vi "Get Ethernet Configuration.vi"(8 "error in (no error)":errorcluster, 11 "Ethernet in":refnum<class "ENET_BS120x.lvclass">) -> (0 "error out":errorcluster, 1 "Configuration Error?":bool, 2 "Ethernet Settings":T1, 3 "Ethernet out":refnum<class "ENET_BS120x.lvclass">)   [LabVIEW 2021, in "BS120x Driver.lvlib" / "ENET_BS120x.lvclass"]
doc: "Retrieve Battery Simulator 1200 Ethernet settings.\n(c) 2019 Bloomy Controls, Inc. All rights reserved."
uses:
  ENET_BS120x.lvclass
  TypeDefs/Ethernet Settings.ctl
  BS120x.lvclass
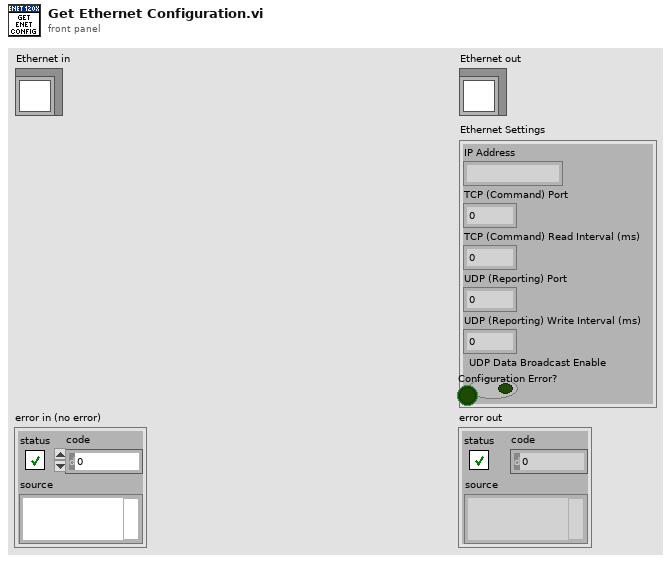
[diagram p1: front panel]
types:
  T1 = typedef "BS120x Driver.lvlib/BS120x.lvclass/Ethernet Settings.ctl" = cluster{"IP Address":string, "TCP (Command) Port":u16, "TCP (Command) Read Interval (ms)":u32, "UDP (Reporting) Port":u16, "UDP (Reporting) Write Interval (ms)":u32, "UDP Data Broadcast Enable":bool}
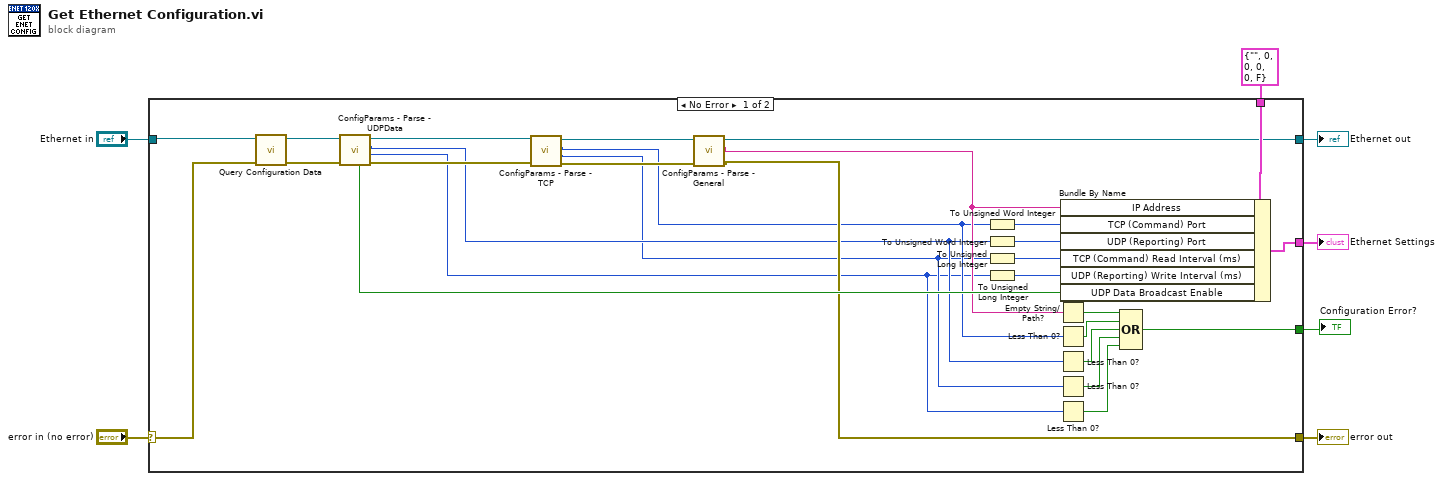
[diagram p0: block diagram]
diagram:
  n1 = case shown="No Error" "error in (no error)" {
    selector: "error in (no error)" -> [w20 w38]
    tunnel: [w14 w38] -> w6
    tunnel: [w13 w37] -> w4
    tunnel: "Ethernet in" -> [w23 w37]
    tunnel: [w34 w36] -> w2
    tunnel: T1 {"IP Address"="", "TCP (Command) Port"=0, "TCP (Command) Read Interval (ms)"=0, "UDP (Reporting) Port"=0, "UDP (Reporting) Write Interval (ms)"=0, "UDP Data Broadcast Enable"=FALSE} ("Ethernet Settings") -> [w35 w36]
    tunnel: [w28 _] -> w1
    frame No Error {
      n2 = call-dynamic "Query Configuration Data.vi"("error in (no error)"=w20, "Ethernet in"=w23) -> ("error out"=w19:errorcluster, "Ethernet out"=w22:refnum<class "ENET_BS120x.lvclass">)  [unwired: 6 in, 2 out]
      n3 = call-dynamic "ConfigParams - Parse - UDPData.vi"("error in (no error)"=w19, "Ethernet in"=w22) -> ("error out"=w18:errorcluster, "UDPDataPeriod_mS"=w8:i32, "UDP Data Port"=w10:i32, "Ethernet out"=w17:refnum<class "ENET_BS120x.lvclass">, "UDP Data Enable"=w21:bool)  [unwired: 5 in]
      n4 = call-dynamic "ConfigParams - Parse - TCP.vi"("error in (no error)"=w18, "Ethernet in"=w17) -> ("error out"=w15:errorcluster, "TCPLoopTime_ms"=w9:i32, "TCPCommandPort"=w11:i32, "Ethernet out"=w16:refnum<class "ENET_BS120x.lvclass">)  [unwired: 6 in]
      n5 = call-dynamic "ConfigParams - Parse - General.vi"("error in (no error)"=w15, "Ethernet in"=w16) -> ("error out"=w14:errorcluster, "IPAddress"=w12:string, "Ethernet out"=w13:refnum<class "ENET_BS120x.lvclass">)  [unwired: 6 in, 1 out]
      n6 = To Unsigned Word Integer(number=w11) -> (unsigned 16bit integer=w27:u16)
      n7 = To Unsigned Word Integer(number=w10) -> (unsigned 16bit integer=w26:u16)
      n8 = To Unsigned Long Integer(number=w9) -> (unsigned 32bit integer=w25:u32)
      n9 = To Unsigned Long Integer(number=w8) -> (unsigned 32bit integer=w24:u32)
      n10 = Empty String/Path?(string/path=w12) -> (empty?=w33:bool)
      n11 = Less Than 0?(x=w11) -> (x < 0?=w32:bool)
      n12 = Less Than 0?(x=w10) -> (x < 0?=w31:bool)
      n13 = Less Than 0?(x=w9) -> (x < 0?=w30:bool)
      n14 = Less Than 0?(x=w8) -> (x < 0?=w29:bool)
      n15 = Bundle By Name(cluster=w35, "IP Address"=w12, "TCP (Command) Port"=w27, "UDP (Reporting) Port"=w26, "TCP (Command) Read Interval (ms)"=w25, "UDP (Reporting) Write Interval (ms)"=w24, "UDP Data Broadcast Enable"=w21) -> (w34:T1)
      n16 = Compound Arithmetic op=OR(w33, w32, w31, w30, w29) -> (w28:bool)
    }
    frame Error {
    }
  }
  "error out" <- w6
  "Ethernet out" <- w4
  "Ethernet Settings" <- w2
  "Configuration Error?" <- w1
